vi "PowerSupplyOscilloscopeBasicReader.vi"() -> ()   [LabVIEW 2020]
uses:
  Oscilloscope/Oscilloscope.lvclass
  PowerSupply/PowerSupply.lvclass
  PowerSupply/PowerSupplyChannelSelection.ctl
  Oscilloscope/Oscilloscope.lvclass/Oscilloscope.ctl
panel:
  in  "Stop Button":bool
  out "Waveform Graph":waveform(dbl)[](graph)
  out "error out":errorcluster
  out "AnalogWaveform":waveform(dbl)[](array[waveform]) caption="Analog Waveforms"
  in  "error in (no error)":errorcluster
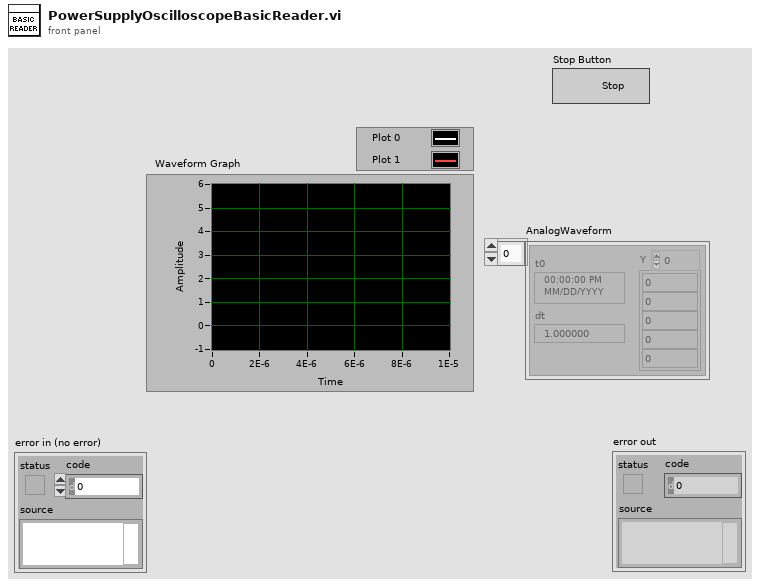
[diagram p1: front panel]
types:
  T1 = typedef "PowerSupplyChannelSelection.ctl" = enum16{"ps/+5V", "ps/-5V"}
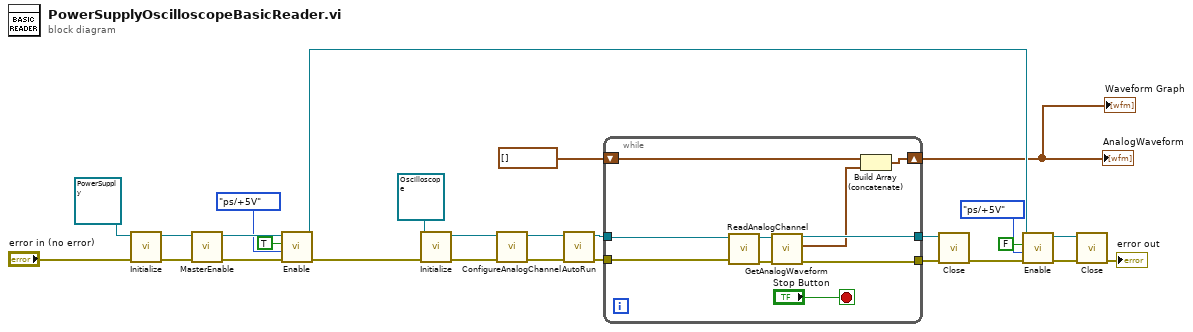
[diagram p0: block diagram]
diagram:
  n1 = call-dynamic "Initialize.vi"("error in (no error)"="error in (no error)", "PowerSupply in"=refnum<class "PowerSupply.lvclass"> refnum) -> ("error out"=w22:errorcluster, "PowerSupply out"=w23:refnum<class "PowerSupply.lvclass">)  [unwired: 8 in]
  n2 = call "MasterEnable.vi"("error in (no error)"=w22, "PowerSupply in"=w23) -> ("error out"=w18:errorcluster, "PowerSupply out"=w21:refnum<class "PowerSupply.lvclass">)  [unwired: 8 in]
  n3 = call "Enable.vi"("error in (no error)"=w18, "ChannelSelection"=PowerSupplyChannelSelection."ps/+5V", "Enable"=TRUE, "PowerSupply in"=w21) -> ("error out"=w16:errorcluster, "PowerSupply out"=w14:refnum<class "PowerSupply.lvclass">)  [unwired: 6 in]
  n4 = call-dynamic "Initialize.vi"("error in (no error)"=w16, "Oscilloscope in"=refnum<class "Oscilloscope.lvclass"> refnum) -> ("error out"=w26:errorcluster, "Oscilloscope out"=w27:refnum<class "Oscilloscope.lvclass">)  [unwired: 8 in]
  n5 = call "ConfigureAnalogChannel.vi"("error in (no error)"=w26, "Oscilloscope in"=w27) -> ("error out"=w1:errorcluster, "Oscilloscope out"=w2:refnum<class "Oscilloscope.lvclass">)  [unwired: 8 in]
  n6 = call "AutoRun.vi"("error in (no error)"=w1, "Oscilloscope in"=w2) -> ("error out"=w3:errorcluster, "Oscilloscope out"=w4:refnum<class "Oscilloscope.lvclass">)  [unwired: 8 in]
  n7 = while {
    tunnel: w4 -> [w35]
    tunnel: [w34] -> w8
    tunnel: [w33] -> w7
    shift-right: [w29] -> w5
    shift-left: waveform(dbl)[] [] ("AnalogWaveform") -> [w31]
    tunnel: w3 -> [w28]
    stop <- "Stop Button" stop-if-true
    n8 = call "ReadAnalogChannel.vi"("error in (no error)"=w28, "Oscilloscope in"=w35) -> ("error out"=w37:errorcluster, "Oscilloscope out"=w36:refnum<class "Oscilloscope.lvclass">)  [unwired: 8 in]
    n9 = call "GetAnalogWaveform.vi"("error in (no error)"=w37, "Oscilloscope in"=w36) -> ("error out"=w34:errorcluster, "AnalogWaveform"=w30:waveform(dbl)[], "Oscilloscope out"=w33:refnum<class "Oscilloscope.lvclass">)  [unwired: 7 in]
    n10 = Build Array (concatenate)(w31, w30) -> (w29:waveform(dbl)[])
  }
  "AnalogWaveform" <- w5
  "Waveform Graph" <- w5
  n11 = call-dynamic "Close.vi"("error in (no error)"=w8, "Oscilloscope in"=w7) -> ("error out"=w13:errorcluster)  [unwired: 8 in, 1 out]
  n12 = call "Enable.vi"("error in (no error)"=w13, "ChannelSelection"=PowerSupplyChannelSelection."ps/+5V", "Enable"=FALSE, "PowerSupply in"=w14) -> ("error out"=w12:errorcluster, "PowerSupply out"=w10:refnum<class "PowerSupply.lvclass">)  [unwired: 6 in]
  n13 = call-dynamic "Close.vi"("error in (no error)"=w12, "PowerSupply in"=w10) -> ("error out"=→"error out":errorcluster)  [unwired: 8 in, 1 out]
